vi "6502 Clock Gen And EEPROM Simulator.vi"() -> ()   [LabVIEW 2021]
uses:
  Disassembler/Addressing Mode.ctl
  Disassembler/Menmonic.ctl
  Disassembler/Disassembler.lvclass
  IO/IO.lvclass/IO.ctl
  Memory/Memory.lvclass/Memory.ctl
  IO/IO.lvclass
  Memory/Memory.lvclass
  Hex Viewer/Hex Viewer.lvclass
panel:
  out "VIA":string[][](table)
  in  "Enable Debug Visualisation":bool
  out "RAM":string[][](table)
  out "EEPROM":string[][](table)
  out "Mnemonic":T1=enum."NOP"
  out "Addressing Mode":T2=enum."Immediate"
  out "Measured Clock Frequency [Hz]":dbl format="%.1p"
  out "R/W":bool
  out "Data":u8 format="%02x"
  out "CLK":bool
  in  "Single Step":bool
  in  "Free Running":bool
  in  "Clock Half Period [ms]":u32
  out "Address":u16 format="%04x"
  # "Clock"
  # "Clock rising edge: setup data\n\nClock falling edge: sample data"
  # "Disassembly"
  # "As no kind of program counter is implemented this will give garbage for all non-instructions that appear on the data bus."
  # "IO"
  # "R/W false: CPU writes to data bus \n\nR/W true: CPU reads from data bus"
  # "Debug"
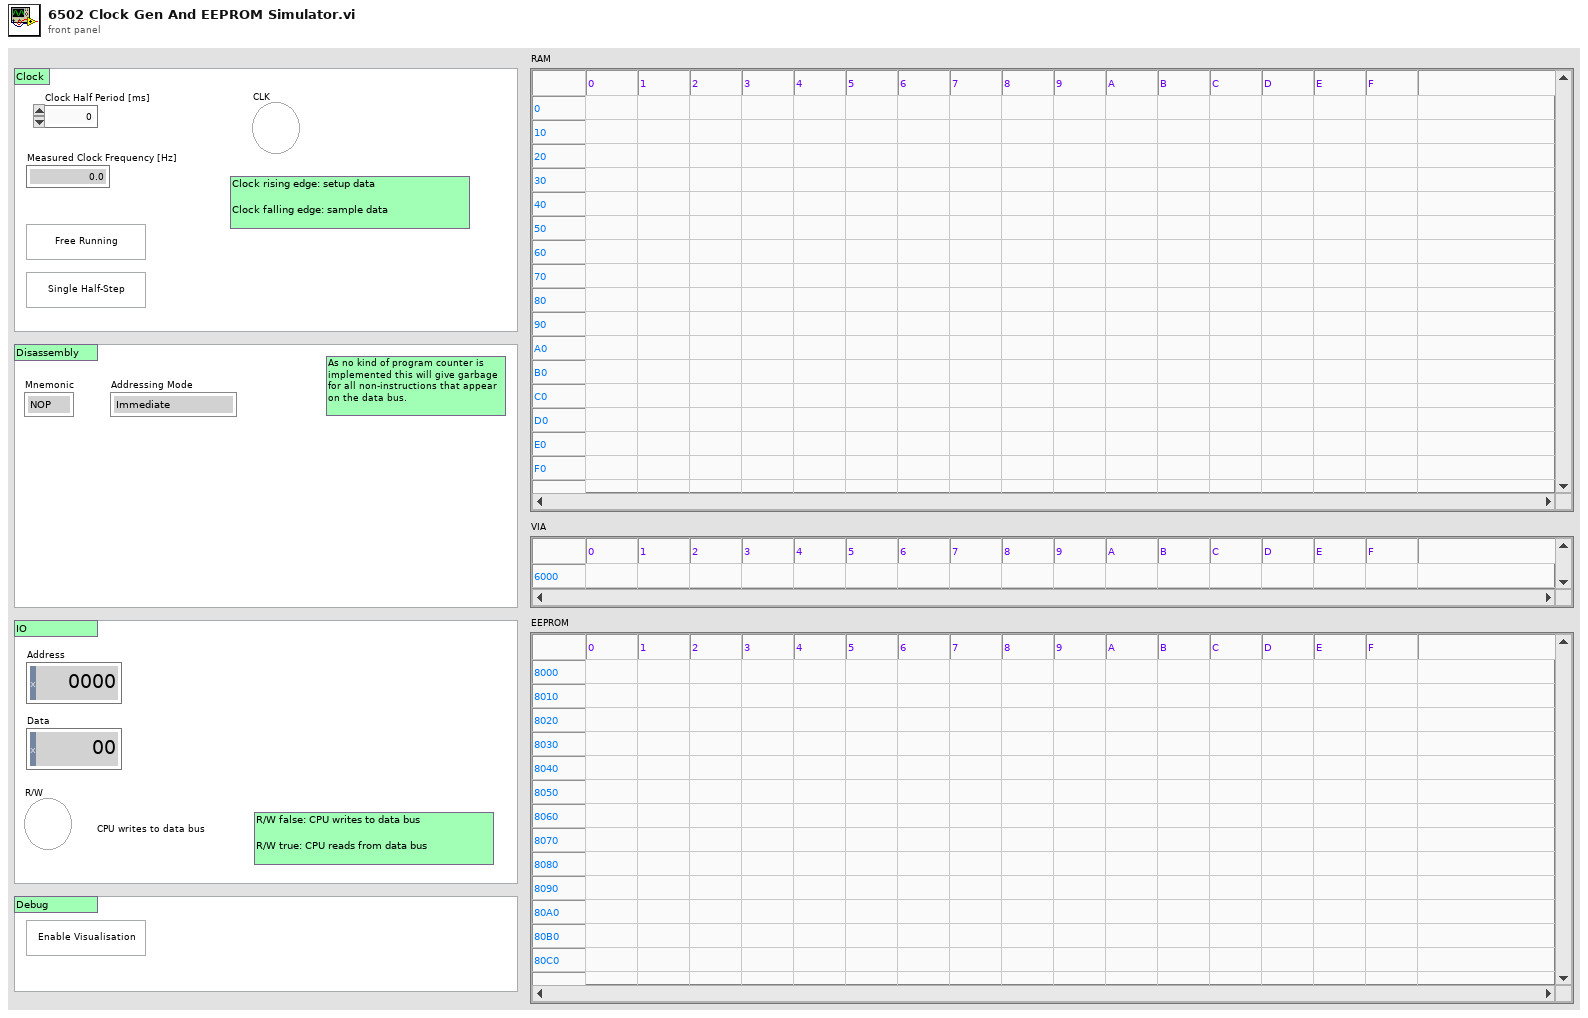
[diagram p1: front panel]
types:
  T1 = typedef "Disassembler.lvclass/Menmonic.ctl" = enum16{"Undefined", "ADC", "AND", "ASL", "BCC", "BCS", "BEQ", "BIT", "BMI", "BNE", "BPL", "BRK", "BVC", "BVS", "CLC", "CLD", "CLI", "CLV", "CMP", "CPX", "CPY", "DEC", "DEX", "DEY", "EOR", "INC", "INX", "INY", "JMP", "JSR", "LDA", "LDX", "LDY", "LSR", "NOP", "ORA", "PHA", "PHP", "PLA", "PLP", "ROL", "ROR", "RTI", "RTS", "SBC", "SEC", "SED", "SEI", "STA", "STX", "STY", "TAX", "TAY", "TSX", "TXA", "TXS", "TYA"}
  T2 = typedef "Disassembler.lvclass/Addressing Mode.ctl" = enum16{"Undefined", "Zero Page,Y", "Zero Page,X", "Zero Page", "Relative", "(indirect,X)", "(indirect),Y", "Implicit", "Immediate", "Accumulator", "Absolute,Y", "Absolute,X", "Absolute", "Indirect"}
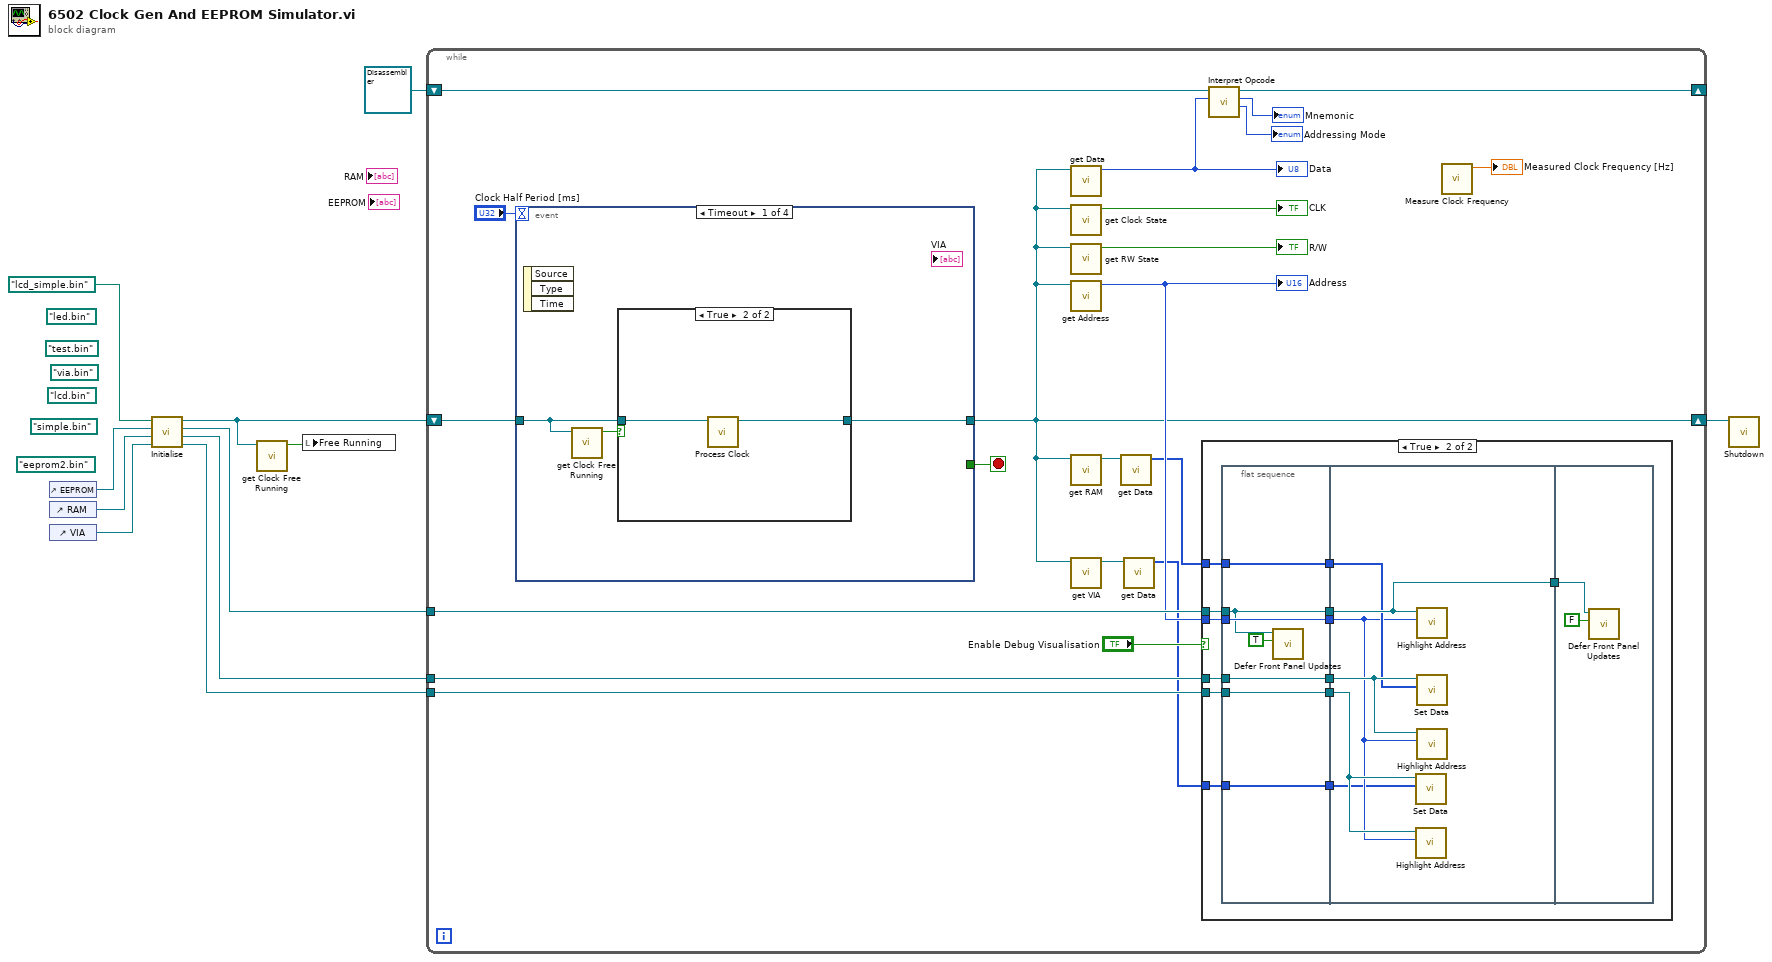
[diagram p0: block diagram]
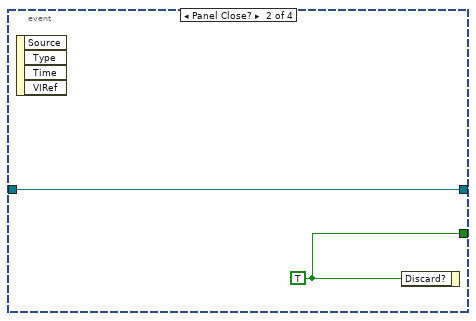
[diagram p4: hidden frame]
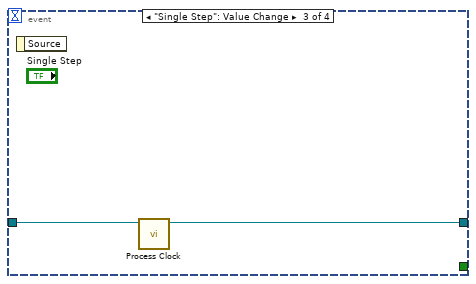
[diagram p5: hidden frame]
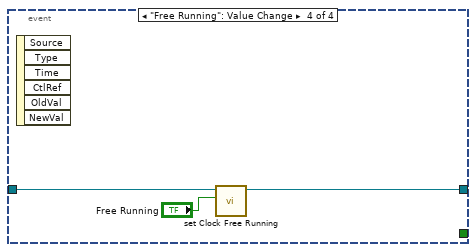
[diagram p6: hidden frame]
diagram:
  (unwired) path "eeprom2.bin" ("ROM")
  (unwired) path "simple.bin" ("ROM")
  (unwired) path "lcd.bin" ("ROM")
  (unwired) path "led.bin" ("ROM")
  (unwired) path "test.bin" ("ROM")
  (unwired) path "via.bin" ("ROM")
  n1 = control-ref of="EEPROM"() -> (w7:refnum<vi>)
  n2 = control-ref of="RAM"() -> (w5:refnum<vi>)
  n3 = control-ref of="VIA"() -> (w3:refnum<vi>)
  n4 = call "Initialise.vi"("VIA"=w3, "RAM"=w5, "EEPROM"=w7, "ROM"=path "lcd_simple.bin") -> ("VIA Viewer"=w2:refnum<class "Hex Viewer.lvclass">, "RAM Viewer"=w4:refnum<class "Hex Viewer.lvclass">, "EEPROM Viewer"=w6:refnum<class "Hex Viewer.lvclass">, "IO out"=w10:refnum<class "IO.lvclass">)  [unwired: 4 in]
  n5 = call "get Clock Free Running.vi"("Clock Generator in"=w10) -> ("Free Running"=w11:bool)  [unwired: 10 in]
  n6 = local write "Free Running"(w11) -> ()
  n7 = while {
    shift-right: [w14] -> w9
    shift-left: w10 -> [w30]
    tunnel: w6 -> [w27]
    tunnel: w4 -> [w26]
    shift-right: [w16] -> _
    shift-left: refnum<class "Disassembler.lvclass"> refnum ("Disassembler.lvclass") -> [w28]
    tunnel: w2 -> [w15]
    stop <- w31 stop-if-true
    n8 = event shown="[0] Timeout" {
      selector: _ -> [_ _ _ _]
      dyn-events: _ -> [_ _ _ _]
      timeout: "Clock Half Period [ms]" -> [_ _ _ _]
      tunnel: [_ w68 _ _] -> w31
      tunnel: w30 -> [w62 w67 w69 w73]
      tunnel: [w63 w67 w70 w72] -> w14
      event Timeout {
        n9 = event-data() -> ()  [unwired: 1 in, 3 out]
        n10 = call "get Clock Free Running.vi"("Clock Generator in"=w62) -> ("Free Running"=w61:bool)  [unwired: 10 in]
        n11 = case shown="True" w61 {
          tunnel: w62 -> [w64 w66]
          tunnel: [w64 w65] -> w63
          frame False {
          }
          frame True {
            n12 = call "Process Clock.vi"("IO in"=w66) -> ("IO out"=w65:refnum<class "IO.lvclass">)  [unwired: 10 in]
          }
        }
      }
      event Panel Close? {
        w68 = TRUE ("Discard?")
        n13 = event-data() -> ()  [unwired: 1 in, 4 out]
        n14 = event-data("Discard?"=w68) -> ()  [unwired: 1 in, 1 out]
      }
      event "Single Step": Value Change {
        n15 = event-data() -> ()  [unwired: 1 in, 1 out]
        n16 = call "Process Clock.vi"("IO in"=w69) -> ("IO out"=w70:refnum<class "IO.lvclass">)  [unwired: 10 in]
      }
      event "Free Running": Value Change {
        n17 = event-data() -> ()  [unwired: 1 in, 6 out]
        n18 = call "set Clock Free Running.vi"("Free Running"="Free Running", "Clock Generator in"=w73) -> ("Clock Generator out"=w72:refnum<class "IO.lvclass">)  [unwired: 9 in]
      }
    }
    n19 = call "get Data.vi"("IO in"=w14) -> ("Data"=w22:u8)  [unwired: 10 in]
    "Data" <- w22
    n20 = call "get Clock State.vi"("Clock Generator in"=w14) -> ("Current State"=→"CLK":bool)  [unwired: 10 in]
    n21 = call "get RW State.vi"("IO in"=w14) -> ("R/W State"=→"R/W":bool)  [unwired: 10 in]
    n22 = call "get Address.vi"("IO in"=w14) -> ("Address"=w19:u16)  [unwired: 10 in]
    "Address" <- w19
    n23 = call "get RAM.vi"("IO in"=w14) -> ("Memory"=w23:refnum<class "Memory.lvclass">)  [unwired: 10 in]
    n24 = call "get VIA.vi"("IO in"=w14) -> ("Memory"=w13:refnum<class "Memory.lvclass">)  [unwired: 10 in]
    n25 = call "get Data.vi"("Memory in"=w23) -> ("Data"=w18:u8[])  [unwired: 10 in]
    n26 = call "get Data.vi"("Memory in"=w13) -> ("Data"=w12:u8[])  [unwired: 10 in]
    n27 = case shown="True" "Enable Debug Visualisation" {
      tunnel: w27 -> [_ w40]
      tunnel: w26 -> [_ w39]
      tunnel: w19 -> [_ w38]
      tunnel: w18 -> [_ w37]
      tunnel: w15 -> [_ w35]
      tunnel: w12 -> [_ w33]
      frame False {
      }
      frame True {
        n28 = flat-sequence {
          tunnel: w39 -> [w51]
          tunnel: w38 -> [w52]
          tunnel: w40 -> [w50]
          tunnel: [w50] -> w45
          tunnel: [w52] -> w44
          tunnel: [w51] -> w43
          tunnel: w37 -> [w48]
          tunnel: [w48] -> w42
          tunnel: [w47] -> w36
          tunnel: w35 -> [w47]
          tunnel: [w46] -> w34
          tunnel: w33 -> [w46]
          tunnel: w45 -> [w57]
          tunnel: w44 -> [w54]
          tunnel: w43 -> [w58]
          tunnel: [w57] -> w41
          tunnel: w42 -> [w56]
          tunnel: w36 -> [w55]
          tunnel: w34 -> [w53]
          tunnel: w41 -> [w60]
          frame #0 {
            n29 = call "Defer Front Panel Updates.vi"("Defer"=TRUE, "Hex Viewer in"=w50) -> ()  [unwired: 9 in, 1 out]
          }
          frame #1 {
            n30 = call "Set Data.vi"("Data"=w53, "Hex Viewer in"=w55) -> ()  [unwired: 9 in, 1 out]
            n31 = call "Highlight Address.vi"("Address"=w54, "Hex Viewer in"=w55) -> ()  [unwired: 10 in]
            n32 = call "Highlight Address.vi"("Address"=w54, "Hex Viewer in"=w57) -> ()  [unwired: 10 in]
            n33 = call "Set Data.vi"("Data"=w56, "Hex Viewer in"=w58) -> ()  [unwired: 9 in, 1 out]
            n34 = call "Highlight Address.vi"("Address"=w54, "Hex Viewer in"=w58) -> ()  [unwired: 10 in]
          }
          frame #2 {
            n35 = call "Defer Front Panel Updates.vi"("Defer"=FALSE, "Hex Viewer in"=w60) -> ()  [unwired: 9 in, 1 out]
          }
        }
      }
    }
    n36 = call "Interpret Opcode.vi"("Opcode"=w22, "Disassembler in"=w28) -> ("Addressing Mode"=→"Addressing Mode":T2, "Mnemonic"=→"Mnemonic":T1, "Disassembler out"=w16:refnum<class "Disassembler.lvclass">)  [unwired: 7 in]
    n37 = call "Measure Clock Frequency.vi"() -> ("Measured Clock Frequence [Hz]"=→"Measured Clock Frequency [Hz]":dbl)  [unwired: 11 in]
  }
  n38 = call "Shutdown.vi"("IO in"=w9) -> ()  [unwired: 11 in]
